vi "Display and Log Process.vi"() -> ()   [LabVIEW 2015, in "VS Inline Async API.lvlib"]
uses:
  VS Inline Async API.lvlib
  Process/Process.lvclass
  Process/Process.lvclass/Process.ctl
  Process/Data Member Access/Read Name.vi
  Process/Data Member Access/Read Process.Trigger.vi
  Process/Data Member Access/Read Process.Stop.vi
  <vilib>/NI Veristand/Custom Device Tools/Custom Device Utility Library/Custom Device Utility Library.lvlib
panel:
  in  "Parameters":variant
  in  "Process":refnum<class "Process.lvclass">
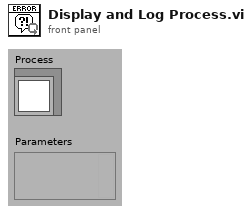
[diagram p1: front panel]
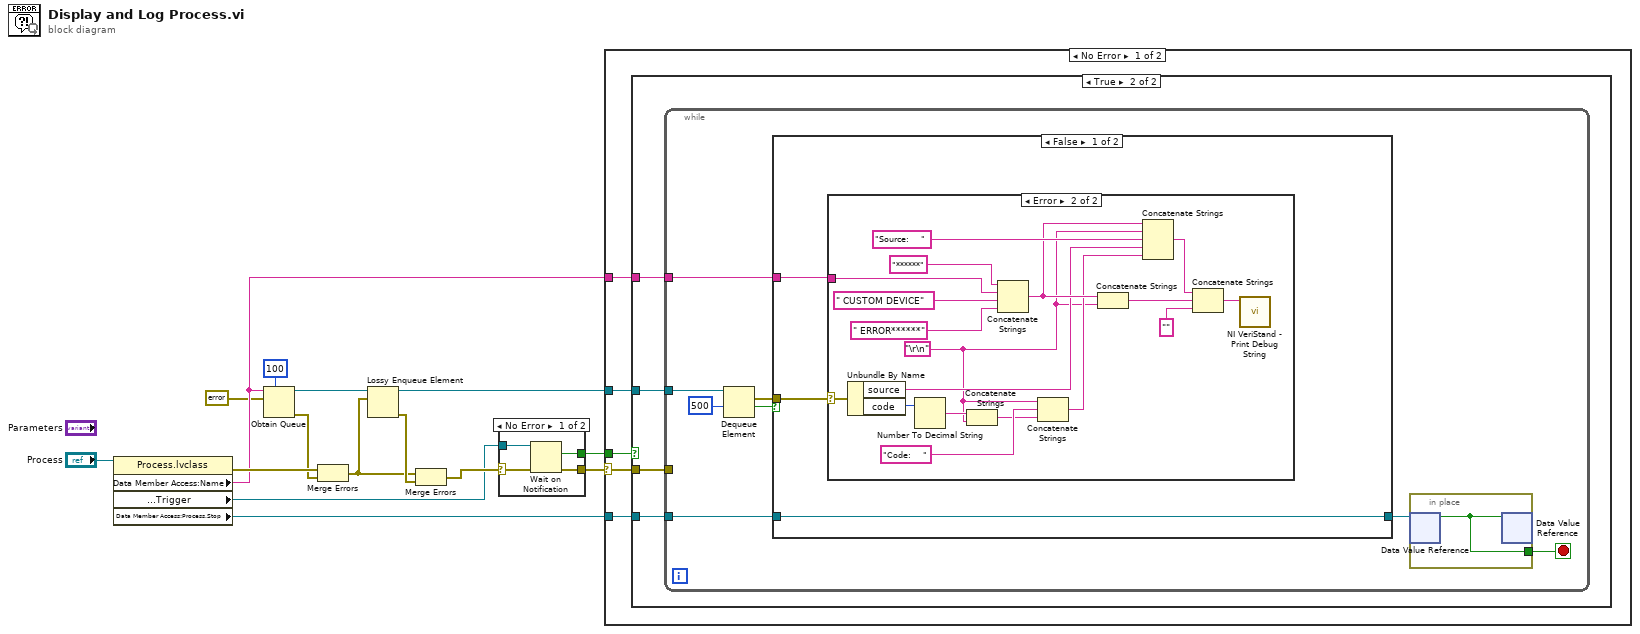
[diagram p0: block diagram]
diagram:
  n1 = property class="Process.lvclass"(reference="Process") -> (error out=w8:errorcluster, "Data Member Access:Name"=w4:string, "Data Member Access:Process.Trigger"=w5:refnum<notifier>, "Data Member Access:Process.Stop"=w11:refnum<data-value>)  [unwired: 1 in, 1 out]
  n2 = Obtain Queue(max queue size (-1, unlimited)=100, name (unnamed)=w4, element data type=errorcluster {"status"=FALSE, "code"=0, "source"=""} ("error out")) -> (queue out=w15:refnum<queue>, error out=w3:errorcluster)  [unwired: 2 in, 1 out]
  n3 = Merge Errors(w8, w3) -> (w1:errorcluster)
  n4 = Lossy Enqueue Element(queue=w15, element=w1) -> (queue out=w10:refnum<queue>, error out=w7:errorcluster)  [unwired: 1 in, 2 out]
  n5 = Merge Errors(w1, w7) -> (w6:errorcluster)
  n6 = case shown="No Error" w6 {
    selector: w6 -> [w17 w20]
    tunnel: [w19 w20] -> w9
    tunnel: [w18 _] -> w12
    tunnel: w5 -> [w16 _]
    frame No Error {
      n7 = Wait on Notification(notifier=w16, error in (no error)=w17) -> (notification=w18:bool, error out=w19:errorcluster)  [unwired: 2 in, 2 out]
    }
    frame Error {
    }
  }
  n8 = case shown="No Error" w9 {
    selector: w9 -> [w21 _]
    tunnel: w12 -> [w25 _]
    tunnel: w4 -> [w24 _]
    tunnel: w10 -> [w23 _]
    tunnel: w11 -> [w22 _]
    frame No Error {
      n9 = case shown="True" w25 {
        tunnel: w23 -> [_ w29]
        tunnel: w24 -> [_ w28]
        tunnel: w21 -> [_ w27]
        tunnel: w22 -> [_ w26]
        frame False {
        }
        frame True {
          n10 = while {
            tunnel: w29 -> [w37]
            tunnel: w28 -> [w36]
            tunnel: w27 -> [_]
            tunnel: w26 -> [w30]
            stop <- w32 stop-if-true
            n11 = Dequeue Element(queue=w37, timeout in ms (-1)=500) -> (element=w35:errorcluster, timed out?=w33:bool)  [unwired: 1 in, 2 out]
            n12 = case shown="False" w33 {
              tunnel: w35 -> [w40 _]
              tunnel: w36 -> [w39 _]
              tunnel: [w41 w60] -> w31
              tunnel: w30 -> [w41 w60]
              frame False {
                n13 = case shown="Error" w40 {
                  selector: w40 -> [_ w59]
                  tunnel: w39 -> [_ w45]
                  frame No Error {
                  }
                  frame Error {
                    w44 = "\r\n"
                    n14 = Unbundle By Name(w59) -> ("source"=w52:string, "code"=w47:i32)
                    n15 = Number To Decimal String(number=w47) -> (decimal integer string=w56:string)  [unwired: 1 in]
                    n16 = Concatenate Strings(w56, w44) -> (w46:string)
                    n17 = Concatenate Strings("******" ("String"), w45, " CUSTOM DEVICE" ("String"), " ERROR******" ("String")) -> (w53:string)
                    n18 = Concatenate Strings(w44, "Code:    " ("String"), w46) -> (w51:string)
                    n19 = Concatenate Strings(w53, w44) -> (w49:string)
                    n20 = Concatenate Strings(w53, w44, "Source:    " ("String"), w52, w51) -> (w50:string)
                    n21 = Concatenate Strings(w50, w49, "" ("Message")) -> (w43:string)
                    n22 = call <vilib>:"NI VeriStand - Print Debug String.vi"("Message"=w43) -> ()  [unwired: 10 in, 1 out]
                  }
                }
              }
              frame True {
              }
            }
            n23 = in-place {
              in-place-border: [w38] -> w32
              n24 = in-place-dvr #1(w31) -> (w38:bool)  [unwired: 1 out]
              n25 = in-place-dvr #1(w38) -> ()  [unwired: 2 out]
            }
          }
        }
      }
    }
    frame Error {
    }
  }
